vi "Driver.vi"(1 "GyroDevRef in":T4 {"Sample Rate" min=0.25 max=100.0 step=0.25}, 2 "Square Inputs":bool, 3 "Gyro Reset":bool, 7 "JoystickDevRef in":T2) -> (4 "GyroDevRef out":T4 {"Sample Rate" min=0.25 max=100.0 step=0.25}, 6 "JoystickDevRef out":T2, 10 "Output":T1)   [LabVIEW 2015]
uses:
  <vilib>/Rock Robotics/WPI/Joystick/WPI_JoystickDevRef.ctl
  <vilib>/Rock Robotics/WPI/Joystick/WPI_JoystickDeviceEnum.ctl
  <vilib>/Rock Robotics/WPI/Gyro/WPI_GyroDevRef.ctl
  <vilib>/Rock Robotics/SystemInterfaces/AI/FPGA_AIChannel.ctl
  <vilib>/Rock Robotics/SystemInterfaces/spilib/spi_bus.ctl
  <vilib>/Rock Robotics/Network Tables/NT Write Numeric Array.vi
  <vilib>/Rock Robotics/Network Tables/NT Write String.vi
  <vilib>/Rock Robotics/Network Tables/NT Write Boolean Array.vi
panel:
  # "Analog"
  # "XRS"
  # "Analog"
  # "XRS"
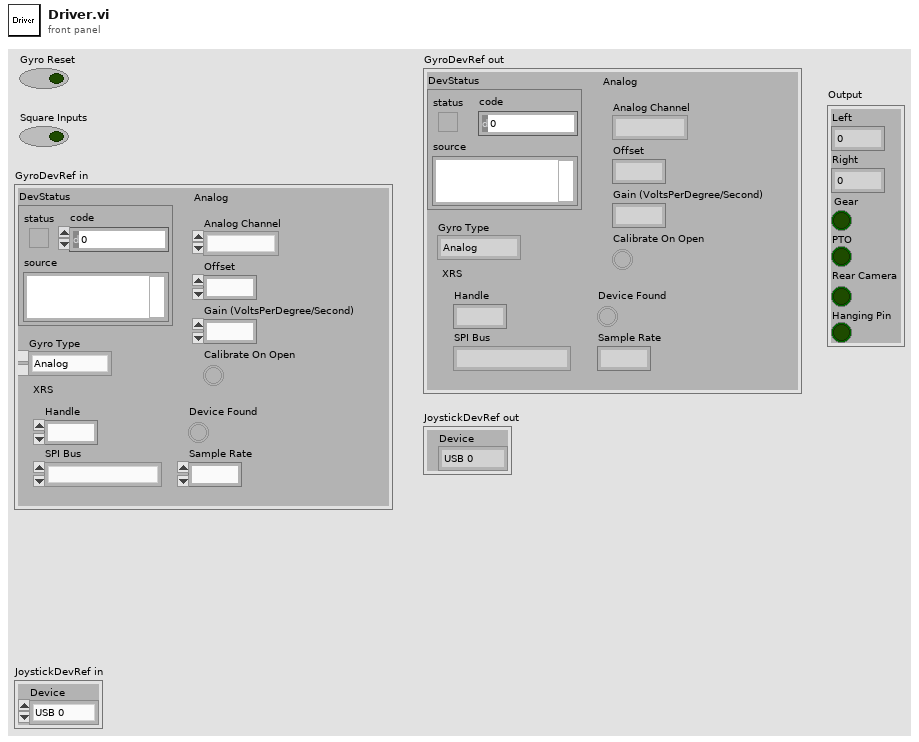
[diagram p1: front panel]
types:
  T1 = cluster{"Left":dbl, "Right":dbl, "Gear":bool, "PTO":bool, "Rear Camera":bool, "Hanging Pin":bool}
  T2 = typedef "WPI_JoystickDevRef.ctl" = cluster{"Device":T3}
  T3 = typedef "WPI_JoystickDeviceEnum.ctl" = enum16{"USB 0", "USB 1", "USB 2", "USB 3", "USB 4", "USB 5"}
  T4 = typedef "WPI_GyroDevRef.ctl" = cluster{"DevStatus":errorcluster, "Analog Channel":T5, "Offset":dbl, "Gain (VoltsPerDegree/Second)":dbl, "Gyro Type":enum16{"Analog", "XRS450"}, "Handle":i32, "SPI Bus":T6, "Device Found":bool, "Sample Rate":dbl, "Calibrate On Open":bool}
  T5 = typedef "FPGA_AIChannel.ctl" = enum8{"AI 0", "AI 1", "AI 2", "AI 3", "AI MXP 0", "AI MXP 1", "AI MXP 2", "AI MXP 3", "Invalid"}
  T6 = typedef "spi_bus.ctl" = enum16{"SPI On-Board, CS0", "SPI On-Board, CS1", "SPI On-Board, CS2", "SPI On-Board, CS3", "SPI MXP", "Invalid"}
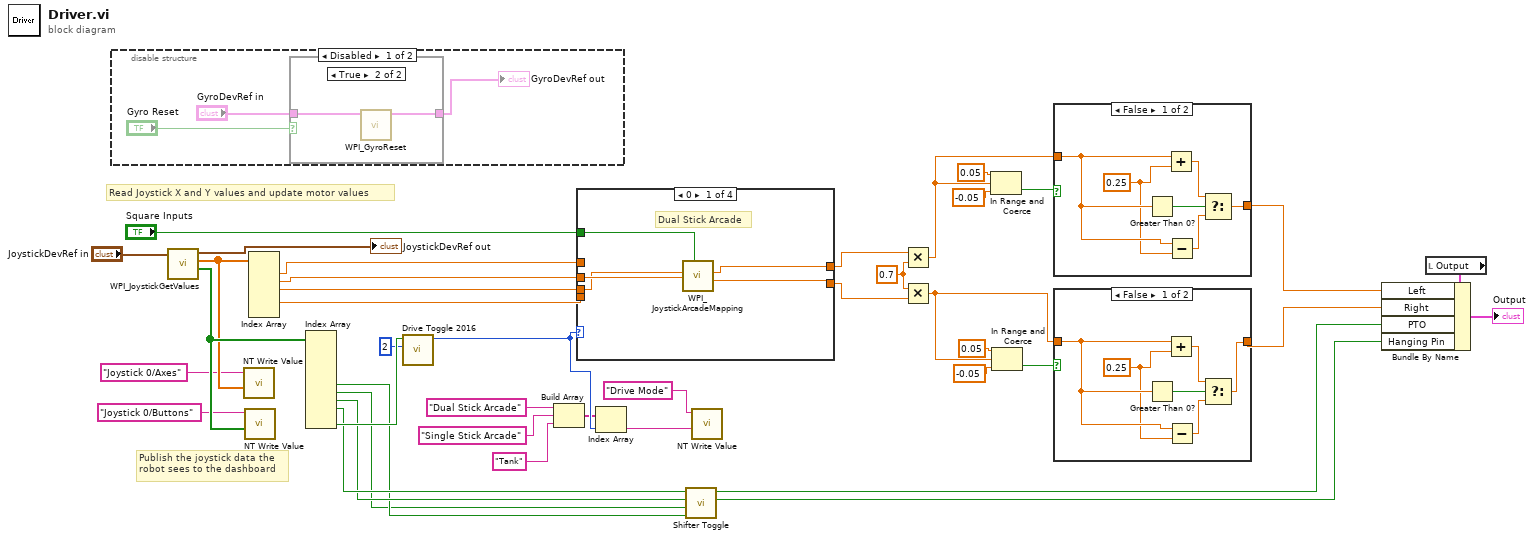
[diagram p0: block diagram]
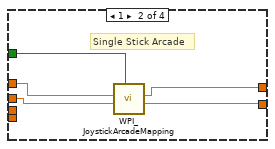
[diagram p6: hidden frame]
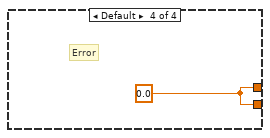
[diagram p8: hidden frame]
diagram:
  w13 = 0.7
  # "Publish the joystick data the\nrobot sees to the dashboard"
  # "Read Joystick X and Y values and update motor values"
  n1 = disable-structure shown="Disabled" {
    frame Disabled {
      n2 = case shown="True" "Gyro Reset" {
        tunnel: "GyroDevRef in" -> [w45 w47]
        tunnel: [w45 w46] -> w43
        frame False {
        }
        frame True {
          n3 = call <vilib>:"WPI_GyroReset.vi"("GyroDevRef"=w47) -> ("GyroDevRef"=w46:T4)  [unwired: 9 in, 1 out]
        }
      }
      "GyroDevRef out" <- w43
    }
    frame Enabled {
    }
  }
  n4 = call <vilib>:"WPI_JoystickGetValues.vi"("JoystickDevRef"="JoystickDevRef in") -> ("Buttons"=w26:bool[], "Axes"=w24:dbl[], "JoystickDevRef"=→"JoystickDevRef out":T2)  [unwired: 6 in, 2 out]
  n5 = call-poly <vilib>:"NT Write Value.vi"("Numeric Array"=w24, "Name"="Joystick 0/Axes") -> ()  [unwired: 9 in, 1 out]
  n6 = call-poly <vilib>:"NT Write Value.vi"("Boolean Array"=w26, "Name"="Joystick 0/Buttons") -> ()  [unwired: 9 in, 1 out]
  n7 = Index Array(array=w24) -> (element #1=w27:dbl, element #2=w28:dbl, element #3=w31:dbl, element #4=w30:dbl)  [unwired: 6 in, 2 out]
  n8 = Index Array(array=w26) -> (element #5=w3:bool, element #6=w1:bool, element #7=w4:bool, element #8=w6:bool, element #10=w37:bool)  [unwired: 10 in, 5 out]
  n9 = call "Drive Toggle 2016.vi"("# of cases"=2 ("Limit"), "Toggle"=w37) -> ("mode switch"=w35:i32)  [unwired: 9 in]
  n10 = Build Array("Dual Stick Arcade", "Single Stick Arcade", "Tank") -> (w33:string[])
  n11 = case shown="0" w35 {
    tunnel: [w52 w57 w58 w60] -> w12
    tunnel: w27 -> [_ w55 _ _]
    tunnel: [w51 w56 w59 w60] -> w11
    tunnel: w28 -> [w49 w54 w58 _]
    tunnel: w30 -> [_ _ w59 _]
    tunnel: w31 -> [w48 _ _ _]
    tunnel: "Square Inputs" -> [w50 w53 _ _]
    frame 0 {
      # "Dual Stick Arcade"
      n12 = call <vilib>:"WPI_JoystickArcadeMapping.vi"("Square Inputs"=w50, "Y axis value"=w49, "X axis value"=w48) -> ("Right Motor Value"=w51:dbl, "Left Motor Value"=w52:dbl)  [unwired: 7 in]
    }
    frame 1 {
      # "Single Stick Arcade"
      n13 = call <vilib>:"WPI_JoystickArcadeMapping.vi"("Square Inputs"=w53, "Y axis value"=w54, "X axis value"=w55) -> ("Right Motor Value"=w56:dbl, "Left Motor Value"=w57:dbl)  [unwired: 7 in]
    }
    frame 2 {
      # "Tank"
    }
    frame Default {
      w60 = 0.0 ("upper limit")
      # "Error"
    }
  }
  n14 = Index Array(array=w33, index=w35) -> (element=w34:string)
  n15 = call "Shifter Toggle.vi"("Pin Out"=w3, "Pin In"=w1, "Drive"=w4, "PTO"=w6) -> ("Pin Status"=w2:bool, "Drive/PTO"=w5:bool)  [unwired: 6 in]
  n16 = call-poly <vilib>:"NT Write Value.vi"("String"=w34, "Name"="Drive Mode") -> ()  [unwired: 9 in, 1 out]
  n17 = Multiply(x=w12, y=w13) -> (x*y=w10:dbl)
  n18 = Multiply(x=w13, y=w11) -> (x*y=w9:dbl)
  n19 = In Range and Coerce(upper limit=0.05, x=w10, lower limit=-0.05) -> (In Range?=w19:bool)  [unwired: 1 out]
  n20 = In Range and Coerce(upper limit=0.05, x=w9, lower limit=-0.05) -> (In Range?=w14:bool)  [unwired: 1 out]
  n21 = case shown="False" w19 {
    tunnel: w10 -> [w62 w67]
    tunnel: [w64 w67] -> w41
    frame False {
      w61 = 0.25 ("y")
      n22 = Greater Than 0?(x=w62) -> (x > 0?=w63:bool)
      n23 = Add(x=w62, y=w61) -> (x+y=w66:dbl)
      n24 = Subtract(x=w62, y=w61) -> (x-y=w65:dbl)
      n25 = Select(t=w66, s=w63, f=w65) -> (s? t:f=w64:dbl)
    }
    frame True {
    }
  }
  n26 = case shown="False" w14 {
    tunnel: w9 -> [w69 w74]
    tunnel: [w71 w74] -> w39
    frame False {
      w68 = 0.25 ("y")
      n27 = Greater Than 0?(x=w69) -> (x > 0?=w70:bool)
      n28 = Add(x=w69, y=w68) -> (x+y=w73:dbl)
      n29 = Subtract(x=w69, y=w68) -> (x-y=w72:dbl)
      n30 = Select(t=w73, s=w70, f=w72) -> (s? t:f=w71:dbl)
    }
    frame True {
    }
  }
  n31 = local read "Output"() -> (w21:T1)
  n32 = Bundle By Name(cluster=w21, "Left"=w41, "Right"=w39, "PTO"=w5, "Hanging Pin"=w2) -> (→"Output":T1)
